vi "ServiceStatusSignals.Create.vi"(8 "error in (no error)":errorcluster, 11 "nodeID in":u64) -> (0 "error out":errorcluster, 3 "nodeID out":u64)   [LabVIEW 2024, in "Diagnostics Addon System Explorer.lvlib"]
uses:
  Diagnostics Addon System Explorer.lvlib
  <vilib>/NI VeriStand/Custom Device API/Custom Device Channel.ctl
  <vilib>/NI VeriStand/Custom Device API/Custom Device Channel Type.ctl
  Addon Shared/SubVIs/Constants.vi
  <vilib>/NI VeriStand/Custom Device API/Custom Device API.lvlib
  Addon Shared/Diagnostics Addon Shared.lvlib
  <vilib>/NI/NI VeriStand Advanced SysDef API/SysDef API/Advanced System Definition.lvlib
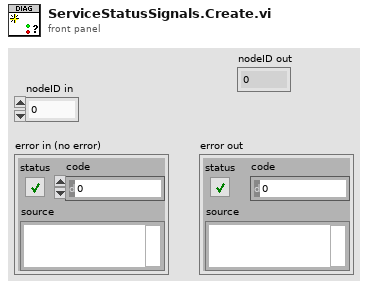
[diagram p1: front panel]
types:
  T1 = typedef "Custom Device API.lvlib/Custom Device Channel.ctl" = cluster{"Type":T2, "Units":string, "Default Value":dbl, "Faultable":bool, "Scalable":bool}
  T2 = typedef "Custom Device API.lvlib/Custom Device Channel Type.ctl" = enum16{"Input", "Output"}
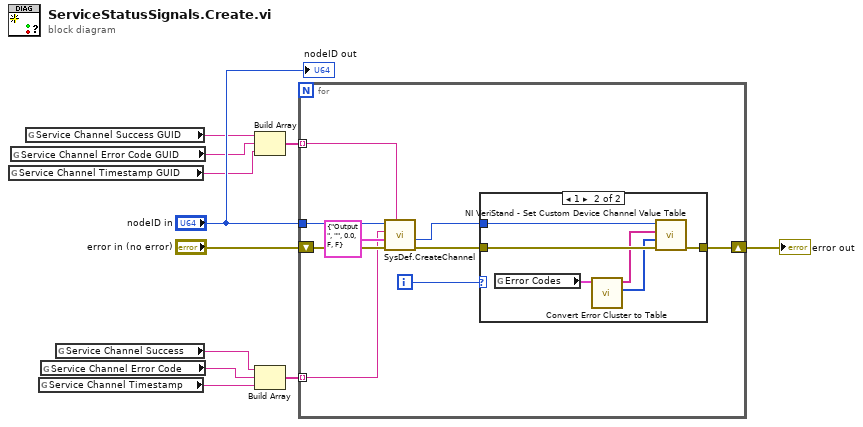
[diagram p0: block diagram]
diagram:
  n1 = global read "Constants.vi" "Service Channel Timestamp GUID"() -> (w3:string)
  n2 = global read "Constants.vi" "Service Channel Error Code GUID"() -> (w4:string)
  n3 = global read "Constants.vi" "Service Channel Success GUID"() -> (w2:string)
  n4 = global read "Constants.vi" "Service Channel Timestamp"() -> (w11:string)
  n5 = global read "Constants.vi" "Service Channel Error Code"() -> (w10:string)
  n6 = global read "Constants.vi" "Service Channel Success"() -> (w9:string)
  n7 = Build Array(w2, w4, w3) -> (w1:string[])
  n8 = Build Array(w9, w10, w11) -> (w7:string[])
  n9 = for {
    tunnel: "nodeID in" -> [w18]
    shift-right: [w13] -> w8
    shift-left: "error in (no error)" -> [w19]
    tunnel: w7 -> [w17] mode=indexing
    tunnel: w1 -> [w12] mode=indexing
    i -> [w16]
    n10 = call <vilib>:"SysDef.CreateChannel.vi"("GUID"=w12, "error in (no error)"=w19, "Channel"=T1 {"Type"=enum."Output", "Units"="", "Default Value"=0.0, "Faultable"=FALSE, "Scalable"=FALSE}, "Name"=w17, "nodeID"=w18) -> ("error out"=w15:errorcluster, "New NodeID"=w14:u64)  [unwired: 3 in, 2 out]
    n11 = case shown="1" w16 {
      tunnel: w15 -> [w21 w26]
      tunnel: w14 -> [_ w27]
      tunnel: [w21 w25] -> w13
      frame 0, Default {
      }
      frame 1 {
        n12 = global read "Constants.vi" "Error Codes"() -> (w22:cluster{"Code":i32, "String":string}[])
        n13 = call "Convert Error Cluster to Table.vi"("Error Codes"=w22) -> ("Code"=w23:i32[], "String"=w24:string[])  [unwired: 9 in]
        n14 = call <vilib>:"NI VeriStand - Set Custom Device Channel Value Table.vi"("error in (no error)"=w26, "Values"=w23, "Names"=w24, "Channel Ref in"=w27) -> ("error out"=w25:errorcluster)  [unwired: 6 in, 1 out]
      }
    }
  }
  "error out" <- w8
  "nodeID out" <- "nodeID in"
